vi "Multiply Rational Polynomials.vi"   [LabVIEW 2020, in "NI_AALPro.lvlib"]
doc: "Multiplies rational polynomial G1 by rational polynomial G2. The data types you wire to the <B>Numerator 1</B>, <B>Denominator 1</B>, <B>Numerator 2</B>, and <B>Denominator 2</B> inputs determine the polymorphic instance to use."
uses:
  <vilib>/Analysis/NI_AALPro.lvlib
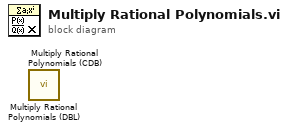
[diagram p0: block diagram]
diagram:
  n1 = call <vilib>:"Multiply Rational Polynomials (DBL).vi"() -> ()  [unwired: 9 in, 3 out]
  n2 = call <vilib>:"Multiply Rational Polynomials (CDB).vi"() -> ()  [unwired: 9 in, 3 out]
